vi "Init Runtime.vi"(8 "error in (no error)":errorcluster, 10 "data allocations":T1, 11 "Sequence Config in":refnum<class "Sequence Config.lvclass">) -> (0 "error out":errorcluster, 2 "Skip":bool, 3 "Sequence Config out":refnum<class "Sequence Config.lvclass">)   [LabVIEW 2015, in "Sequence Config.lvclass"]
uses:
  Sequence Config.lvclass
  <vilib>/NI/Tag Bus Module Framework/channel/data tables.ctl
  <vilib>/NI/Tag Bus/dictionary/data dictionary.lvclass
  <vilib>/NI/Tag Bus/dictionary table pair.ctl
  <vilib>/NI/Tag Bus/table/data table.ctl
  Execution/Sequence.lvclass
  Step/Execution/Step.lvclass
  Step/Config/Step Config.lvclass
  <vilib>/NI/Tag Bus/table/data table.lvlib
  <vilib>/NI/Tag Bus/tag bus.lvlib
  <vilib>/NI/Tag Bus Module Framework/channel/TBM channel.lvclass
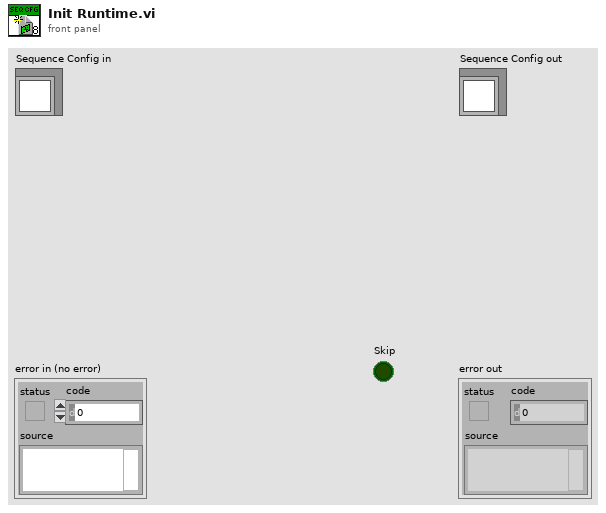
[diagram p1: front panel]
types:
  T1 = typedef "TBM channel.lvclass/data tables.ctl" = cluster{"input data":T2, "processing parameter":T2, "processing result":T2, "output data":T2}
  T2 = typedef "tag bus.lvlib/dictionary table pair.ctl" = cluster{"data dictionary":refnum<class "data dictionary.lvclass">, "data table":T3}
  T3 = typedef "tag bus.lvlib/data table.lvlib/data table.ctl" = cluster{"Double":dbl[], "Single":sgl[], "I64":i64[], "I32":i32[], "I16":i16[], "I8":i8[], "U64":u64[], "U32":u32[], "U16":u16[], "U8":u8[], "Boolean":bool[], "String":string[], "Array of Double":cluster{"DBL Array":dbl[]}[], "Array of Single":cluster{"SGL Array":sgl[]}[], "Array of I64":cluster{"I64 Array":i64[]}[], "Array of I32":cluster{"I32 Array":i32[]}[], "Array of I16":cluster{"I16 Array":i16[]}[], "Array of I8":cluster{"I8 Array":i8[]}[], "Array of U64":cluster{"U64 Array":u64[]}[], "Array of U32":cluster{"U32 Array":u32[]}[], "Array of U16":cluster{"U16 Array":u16[]}[], "Array of U8":cluster{"U8 Array":u8[]}[], "Array of Boolean":cluster{"Boolean Array":bool[]}[], "Array of String":cluster{"String Array":string[]}[]}
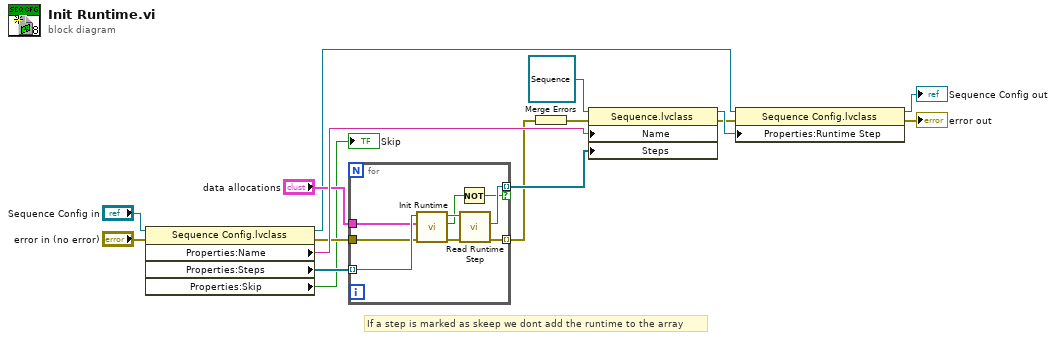
[diagram p0: block diagram]
diagram:
  # "If a step is marked as skeep we dont add the runtime to the array"
  n1 = property class="Sequence Config.lvclass"(reference="Sequence Config in", error in="error in (no error)") -> (reference out=w6:refnum<class "Sequence Config.lvclass">, error out=w4:errorcluster, "Properties:Name"=w13:string, "Properties:Steps"=w16:refnum<class "Step Config.lvclass">[], "Properties:Skip"=→"Skip":bool)
  n2 = for {
    tunnel: w16 -> [w24] mode=indexing
    tunnel: [w25] -> w14 mode=indexing if=w18
    tunnel: "data allocations" -> [w22]
    tunnel: w4 -> [w21]
    tunnel: [w19] -> w12 mode=indexing
    n3 = call-dynamic "Init Runtime.vi"("error in (no error)"=w21, "data allocations"=w22, "Step Config in"=w24) -> ("error out"=w20:errorcluster, "Skip"=w17:bool, "Step Config out"=w23:refnum<class "Step Config.lvclass">)  [unwired: 6 in]
    n4 = Not(x=w17) -> (.not. x?=w18:bool)
    n5 = call-dynamic "Read Runtime Step.vi"("error in (no error)"=w20, "Step Config in"=w23) -> ("error out"=w19:errorcluster, "Step.lvclass"=w25:refnum<class "Step.lvclass">)  [unwired: 7 in, 1 out]
  }
  n6 = Merge Errors(w12) -> (w11:errorcluster)
  n7 = property class="Sequence.lvclass"(reference=refnum<class "Sequence.lvclass"> refnum ("Sequence.lvclass"), error in=w11, "Name"=w13, "Steps"=w14) -> (reference out=w8:refnum<class "Sequence.lvclass">, error out=w1:errorcluster)
  n8 = property class="Sequence Config.lvclass"(reference=w6, error in=w1, "Properties:Runtime Step"=w8) -> (reference out=→"Sequence Config out":refnum<class "Sequence Config.lvclass">, error out=→"error out":errorcluster)
